vi "adreestar.vi"(9 "M+N*8":i32, 10 "ADStatus":i32[](array[numeric]), 11 "ddrlength":i32) -> (3 "adree":i32)   [LabVIEW 2012]
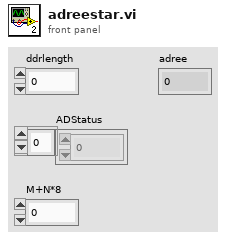
[diagram p1: front panel]
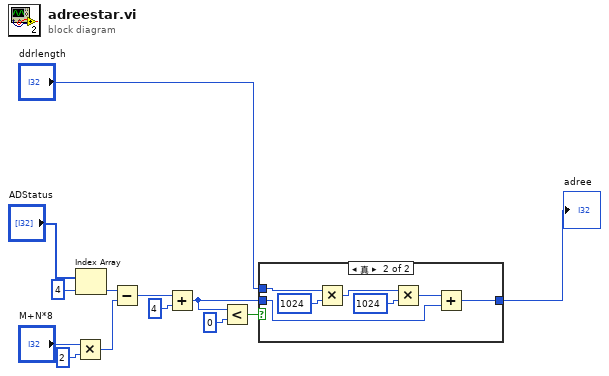
[diagram p0: block diagram]
diagram:
  n1 = Multiply(x="M+N*8", y=2 ("element")) -> (x*y=w5:i32)
  n2 = Index Array(array="ADStatus", index=4 ("element")) -> (element=w9:i32)
  n3 = Subtract(x=w9, y=w5) -> (x-y=w6:i32)
  n4 = Add(x=w6, y=4 ("element")) -> (x+y=w8:i32)
  n5 = Less?(x=w8, y=0) -> (x < y?=w11:bool)
  n6 = case shown="真" w11 {
    tunnel: w8 -> [w14 w17]
    tunnel: [w14 w16] -> w1
    tunnel: "ddrlength" -> [_ w15]
    frame False {
    }
    frame True {
      n7 = Multiply(x=w15, y=1024) -> (x*y=w20:i32)
      n8 = Multiply(x=w20, y=1024) -> (x*y=w18:i32)
      n9 = Add(x=w18, y=w17) -> (x+y=w16:i32)
    }
  }
  "adree" <- w1
